vi "NI_controller_Rel_move_Single Axis.vi"(6 "Initialize":bool, 7 "Velocity (10000)":i32=5000 min=-20000000 max=20000000, 8 "Axis":u16(ring)=2 items=["X axis", "Y axis", "Z axis"], 9 "Relative motion (mm)":dbl=0.02, 10 "Motion ID":T2=1 min=1 max=32 step=1, 11 "Motion System":T1=enum."No Motion Card") -> (0 "Stop position":dbl, 1 "Start Position (mm)":dbl, 3 "Bd ID Out":T3)   [LabVIEW 2022 SP3]
uses:
  <vilib>/Motion/FlexMotion/CustomControls/CustomControls.llb/AxisOrVectorSpace To Configure.flx
  <vilib>/Motion/FlexMotion/FunctionsVIs/StartStopMotion.llb/Start Motion (8 axes).flx
  <vilib>/Motion/FlexMotion/FunctionsVIs/Trajectory.llb/Check Move Complete Status (8 axes).flx
  -NI_MotionRoutines/MotionSys.ctl
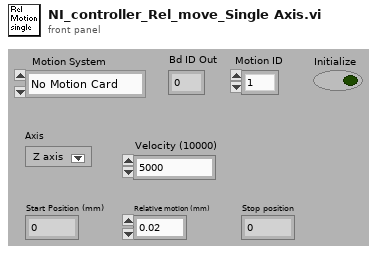
[diagram p1: front panel]
types:
  T1 = typedef "MotionSys.ctl" = enum16{"MM3000", "NI 735x", "Newport ESP", "No Motion Card", "Galil"}
  T2 = typedef "Board Id" = u8
  T3 = typedef "Bd Id Out" = u8
  T4 = enum16{"Absolute Position", "Relative Position", "Velocity", "Relative to Cap Pos", "Modulus Position", "Absolute Contouring", "Relative Contouring"}
  T5 = typedef "AxisOrVectorSpace To Configure.flx" = u16
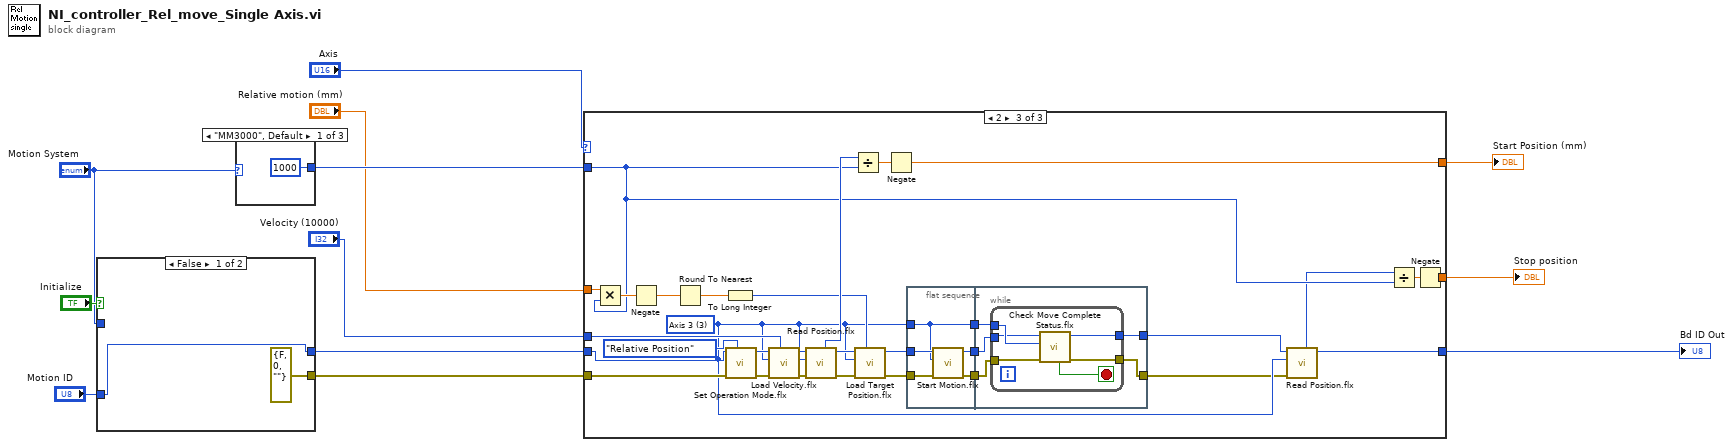
[diagram p0: block diagram]
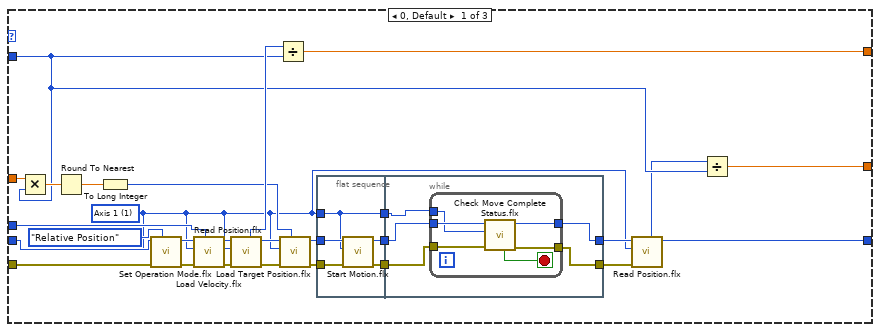
[diagram p2: hidden frame]
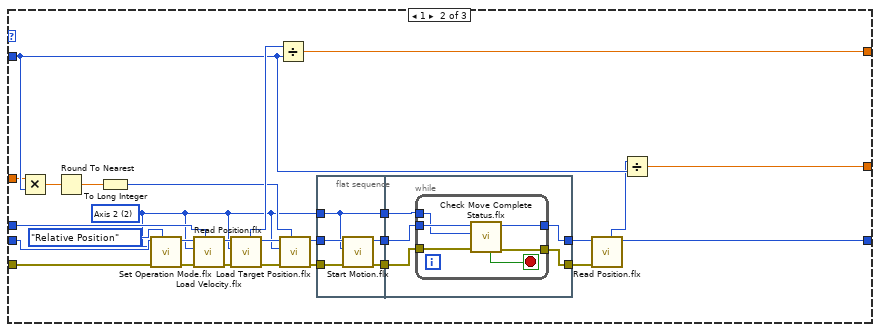
[diagram p3: hidden frame]
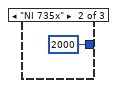
[diagram p4: hidden frame]
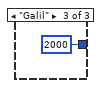
[diagram p5: hidden frame]
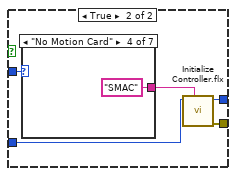
[diagram p6: hidden frame]
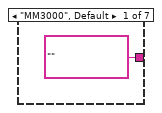
[diagram p7: hidden frame]
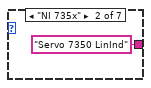
[diagram p8: hidden frame]
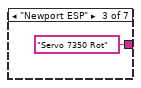
[diagram p9: hidden frame]
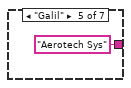
[diagram p10: hidden frame]
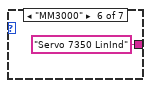
[diagram p11: hidden frame]
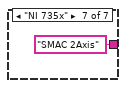
[diagram p12: hidden frame]
diagram:
  n1 = case shown="False" "Initialize" {
    tunnel: [w14 w19] -> w8
    tunnel: [errorcluster {"status"=FALSE, "code"=0, "source"=""} ("error out") w18] -> w7
    tunnel: "Motion ID" -> [w14 w16]
    tunnel: "Motion System" -> [_ w15]
    frame False {
    }
    frame True {
      n2 = case shown="\"No Motion Card\"" w15 {
        tunnel: ["" "Servo 7350 LinInd" "Servo 7350 Rot" "SMAC" "Aerotech Sys" "Servo 7350 LinInd" "SMAC 2Axis"] -> w17
        frame "MM3000", Default {
        }
        frame "NI 735x" {
        }
        frame "Newport ESP" {
        }
        frame "No Motion Card" {
        }
        frame "Galil" {
        }
        frame "MM3000" {
        }
        frame "NI 735x" {
        }
      }
      n3 = call <vilib>:"Initialize Controller.flx"("Settings Name"=w17, "Board ID"=w16) -> ("error out"=w18:errorcluster, "Bd ID Out"=w19:T3)  [unwired: 1 in, 5 out]
    }
  }
  n4 = case shown="\"MM3000\", Default" "Motion System" {
    tunnel: [1000 ("y") 2000 ("y") 2000 ("y")] -> w5
    frame "MM3000", Default {
    }
    frame "NI 735x" {
    }
    frame "Galil" {
    }
  }
  n5 = case shown="2" "Axis" {
    tunnel: w8 -> [w53 w97 w144]
    tunnel: w7 -> [w52 w96 w143]
    tunnel: "Velocity (10000)" -> [w50 w94 w141]
    tunnel: w5 -> [w36 w79 w133]
    tunnel: [w32 w77 w124] -> w4
    tunnel: [w34 w75 w130] -> w3
    tunnel: [w33 w76 w128] -> w2
    tunnel: "Relative motion (mm)" -> [w30 w74 w127]
    frame 0, Default {
      w31 = T5 1 items=["Axis 1"=1, "Axis 2"=2, "Axis 3"=3, "Axis 4"=4, "Axis 5"=5, "Axis 6"=6, "Axis 7"=7, "Axis 8"=8, "Vector Space 1"=17, "Vector Space 2"=18, "Vector Space 3"=19, "Vector Space 4"=20] ("Axis or Vector Space")
      n6 = Multiply(x=w30, y=w36) -> (x*y=w46:dbl)
      n7 = Round To Nearest(number=w46) -> (nearest integer value=w45:dbl)
      n8 = To Long Integer(number=w45) -> (32bit integer=w44:i32)
      n9 = call <vilib>:"Set Operation Mode.flx"("Position Mode (Absolute)"=T4."Relative Position", "error in (no error)"=w52, "Axis or Vector Space"=w31, "Board ID"=w53) -> ("error out"=w55:errorcluster, "Bd ID Out"=w54:T3)  [unwired: 3 out]
      n10 = call <vilib>:"Load Velocity.flx"("Velocity (10000)"=w50, "error in (no error)"=w55, "Axis or Vector Space"=w31, "Board ID"=w54) -> ("error out"=w57:errorcluster, "Bd ID Out"=w56:T3)  [unwired: 4 out]
      n11 = call <vilib>:"Read Position.flx"("error in (no error)"=w57, "Axis"=w31, "Board ID"=w56) -> ("error out"=w47:errorcluster, "Bd ID Out"=w48:T3, "Position"=w49:i32)  [unwired: 4 out]
      n12 = Divide(x=w49, y=w36) -> (x/y=w34:dbl)
      n13 = call <vilib>:"Load Target Position.flx"("Target Position (0)"=w44, "error in (no error)"=w47, "Axis"=w31, "Board ID"=w48) -> ("error out"=w43:errorcluster, "Bd ID Out"=w42:T3)  [unwired: 4 out]
      n14 = flat-sequence {
        tunnel: w43 -> [w62]
        tunnel: w31 -> [w58]
        tunnel: w42 -> [w61]
        tunnel: [w60] -> w41
        tunnel: [w59] -> w40
        tunnel: [w58] -> w37
        tunnel: [w63] -> w39
        tunnel: w41 -> [w66]
        tunnel: [w64] -> w38
        tunnel: w40 -> [w65]
        tunnel: w37 -> [w67]
        frame #0 {
          n15 = call-poly <vilib>:"Start Motion.flx"("error in (no error)"=w62, "Axis or Vector Space"=w58, "Board ID"=w61) -> ("error out"=w59:errorcluster, "Bd ID Out"=w60:T3)  [unwired: 1 in, 3 out]
        }
        frame #1 {
          n16 = while {
            tunnel: w65 -> [w73]
            tunnel: [w72] -> w64
            tunnel: w66 -> [w71]
            tunnel: w67 -> [w70]
            tunnel: [w69] -> w63
            stop <- w68 stop-if-true
            n17 = call-poly <vilib>:"Check Move Complete Status.flx"("error in (no error)"=w73, "Axis or Vector Space"=w70, "Board ID"=w71) -> ("error out"=w72:errorcluster, "Bd ID Out"=w69:T3, "Move Complete"=w68:bool)  [unwired: 1 in, 3 out]
          }
        }
      }
      n18 = call <vilib>:"Read Position.flx"("error in (no error)"=w38, "Axis"=w31, "Board ID"=w39) -> ("Bd ID Out"=w32:T3, "Position"=w35:i32)  [unwired: 5 out]
      n19 = Divide(x=w35, y=w36) -> (x/y=w33:dbl)
    }
    frame 1 {
      w86 = T5 2 items=["Axis 1"=1, "Axis 2"=2, "Axis 3"=3, "Axis 4"=4, "Axis 5"=5, "Axis 6"=6, "Axis 7"=7, "Axis 8"=8, "Vector Space 1"=17, "Vector Space 2"=18, "Vector Space 3"=19, "Vector Space 4"=20] ("Axis or Vector Space")
      n20 = Multiply(x=w74, y=w79) -> (x*y=w90:dbl)
      n21 = Round To Nearest(number=w90) -> (nearest integer value=w89:dbl)
      n22 = To Long Integer(number=w89) -> (32bit integer=w88:i32)
      n23 = call <vilib>:"Set Operation Mode.flx"("Position Mode (Absolute)"=T4."Relative Position", "error in (no error)"=w96, "Axis or Vector Space"=w86, "Board ID"=w97) -> ("error out"=w99:errorcluster, "Bd ID Out"=w98:T3)  [unwired: 3 out]
      n24 = call <vilib>:"Load Velocity.flx"("Velocity (10000)"=w94, "error in (no error)"=w99, "Axis or Vector Space"=w86, "Board ID"=w98) -> ("error out"=w101:errorcluster, "Bd ID Out"=w100:T3)  [unwired: 4 out]
      n25 = call <vilib>:"Read Position.flx"("error in (no error)"=w101, "Axis"=w86, "Board ID"=w100) -> ("error out"=w91:errorcluster, "Bd ID Out"=w92:T3, "Position"=w93:i32)  [unwired: 4 out]
      n26 = Divide(x=w93, y=w79) -> (x/y=w75:dbl)
      n27 = call <vilib>:"Load Target Position.flx"("Target Position (0)"=w88, "error in (no error)"=w91, "Axis"=w86, "Board ID"=w92) -> ("error out"=w87:errorcluster, "Bd ID Out"=w85:T3)  [unwired: 4 out]
      n28 = flat-sequence {
        tunnel: w87 -> [w106]
        tunnel: w86 -> [w102]
        tunnel: w85 -> [w105]
        tunnel: [w104] -> w84
        tunnel: [w103] -> w83
        tunnel: [w102] -> w80
        tunnel: [w110] -> w82
        tunnel: w84 -> [w109]
        tunnel: [w111] -> w81
        tunnel: w83 -> [w107]
        tunnel: w80 -> [w108]
        frame #0 {
          n29 = call-poly <vilib>:"Start Motion.flx"("error in (no error)"=w106, "Axis or Vector Space"=w102, "Board ID"=w105) -> ("error out"=w103:errorcluster, "Bd ID Out"=w104:T3)  [unwired: 1 in, 3 out]
        }
        frame #1 {
          n30 = while {
            tunnel: w107 -> [w117]
            tunnel: [w116] -> w111
            tunnel: w109 -> [w115]
            tunnel: w108 -> [w114]
            tunnel: [w113] -> w110
            stop <- w112 stop-if-true
            n31 = call-poly <vilib>:"Check Move Complete Status.flx"("error in (no error)"=w117, "Axis or Vector Space"=w114, "Board ID"=w115) -> ("error out"=w116:errorcluster, "Bd ID Out"=w113:T3, "Move Complete"=w112:bool)  [unwired: 1 in, 3 out]
          }
        }
      }
      n32 = call <vilib>:"Read Position.flx"("error in (no error)"=w81, "Board ID"=w82) -> ("Bd ID Out"=w77:T3, "Position"=w78:i32)  [unwired: 1 in, 5 out]
      n33 = Divide(x=w78, y=w79) -> (x/y=w76:dbl)
    }
    frame 2 {
      w125 = T5 3 items=["Axis 1"=1, "Axis 2"=2, "Axis 3"=3, "Axis 4"=4, "Axis 5"=5, "Axis 6"=6, "Axis 7"=7, "Axis 8"=8, "Vector Space 1"=17, "Vector Space 2"=18, "Vector Space 3"=19, "Vector Space 4"=20] ("Axis or Vector Space")
      n34 = Multiply(x=w127, y=w133) -> (x*y=w138:dbl)
      n35 = Negate(x=w138) -> (-x=w132:dbl)
      n36 = Round To Nearest(number=w132) -> (nearest integer value=w137:dbl)
      n37 = To Long Integer(number=w137) -> (32bit integer=w136:i32)
      n38 = call <vilib>:"Set Operation Mode.flx"("Position Mode (Absolute)"=T4."Relative Position", "error in (no error)"=w143, "Axis or Vector Space"=w125, "Board ID"=w144) -> ("error out"=w146:errorcluster, "Bd ID Out"=w145:T3)  [unwired: 3 out]
      n39 = call <vilib>:"Load Velocity.flx"("Velocity (10000)"=w141, "error in (no error)"=w146, "Axis or Vector Space"=w125, "Board ID"=w145) -> ("error out"=w148:errorcluster, "Bd ID Out"=w147:T3)  [unwired: 4 out]
      n40 = call <vilib>:"Read Position.flx"("error in (no error)"=w148, "Axis"=w125, "Board ID"=w147) -> ("error out"=w139:errorcluster, "Bd ID Out"=w126:T3, "Position"=w140:i32)  [unwired: 4 out]
      n41 = Divide(x=w140, y=w133) -> (x/y=w131:dbl)
      n42 = call <vilib>:"Load Target Position.flx"("Target Position (0)"=w136, "error in (no error)"=w139, "Axis"=w125, "Board ID"=w126) -> ("error out"=w135:errorcluster, "Bd ID Out"=w134:T3)  [unwired: 4 out]
      n43 = Negate(x=w131) -> (-x=w130:dbl)
      n44 = flat-sequence {
        tunnel: w135 -> [w153]
        tunnel: w125 -> [w150]
        tunnel: w134 -> [w152]
        tunnel: [w151] -> w120
        tunnel: [w150] -> w119
        tunnel: [w149] -> w118
        tunnel: w120 -> [w158]
        tunnel: w119 -> [w157]
        tunnel: [w156] -> w122
        tunnel: [w155] -> w121
        tunnel: w118 -> [w154]
        frame #0 {
          n45 = call-poly <vilib>:"Start Motion.flx"("error in (no error)"=w153, "Axis or Vector Space"=w150, "Board ID"=w152) -> ("error out"=w149:errorcluster, "Bd ID Out"=w151:T3)  [unwired: 1 in, 3 out]
        }
        frame #1 {
          n46 = while {
            tunnel: w154 -> [w162]
            tunnel: w158 -> [w163]
            tunnel: w157 -> [w164]
            tunnel: [w161] -> w156
            tunnel: [w160] -> w155
            stop <- w159 stop-if-true
            n47 = call-poly <vilib>:"Check Move Complete Status.flx"("error in (no error)"=w162, "Axis or Vector Space"=w164, "Board ID"=w163) -> ("error out"=w161:errorcluster, "Bd ID Out"=w160:T3, "Move Complete"=w159:bool)  [unwired: 1 in, 3 out]
          }
        }
      }
      n48 = call <vilib>:"Read Position.flx"("error in (no error)"=w122, "Axis"=w125, "Board ID"=w121) -> ("Bd ID Out"=w124:T3, "Position"=w123:i32)  [unwired: 5 out]
      n49 = Divide(x=w123, y=w133) -> (x/y=w129:dbl)
      n50 = Negate(x=w129) -> (-x=w128:dbl)
    }
  }
  "Bd ID Out" <- w4
  "Start Position (mm)" <- w3
  "Stop position" <- w2
